vi "Lab Panel V4.90.vi"() -> ()   [LabVIEW 2013] (continued)
                n1776 = property on="O/I  LAB04-2" class="Bool (strict)"("DisabledEnum"=w3325) -> ()  [unwired: 2 in, 2 out]
                n1777 = property on="O/I  LAB03-2" class="Bool (strict)"("DisabledEnum"=w3327) -> ()  [unwired: 2 in, 2 out]
                n1778 = Not(x=w3332) -> (.not. x?=w3333:bool)
                n1779 = Not(x=w3331) -> (.not. x?=w3334:bool)
                n1780 = Not(x=w3330) -> (.not. x?=w3335:bool)
                n1781 = property on="RESULT LAB05-2" class="Bool (strict)"("Visible"=w3333) -> ()  [unwired: 2 in, 2 out]
                n1782 = property on="RESULT LAB05-1" class="Bool (strict)"("Visible"=w3334) -> ()  [unwired: 2 in, 2 out]
                n1783 = Not(x=w3329) -> (.not. x?=w3336:bool)
                n1784 = property on="RESULT LAB04-2" class="Bool (strict)"("Visible"=w3335) -> ()  [unwired: 2 in, 2 out]
                n1785 = Not(x=w3328) -> (.not. x?=w3337:bool)
                n1786 = property on="RESULT LAB04-1" class="Bool (strict)"("Visible"=w3336) -> ()  [unwired: 2 in, 2 out]
                n1787 = property on="RESULT LAB03-2" class="Bool (strict)"("Visible"=w3337) -> ()  [unwired: 2 in, 2 out]
              }
              frame #2 {
                # "disable calibrate if any test running"
                n1788 = Or(x=w3360, y=w3359) -> (x .or. y?=w3353:bool)
                n1789 = Or(x=w3362, y=w3361) -> (x .or. y?=w3355:bool)
                n1790 = Or(x=w3366, y=w3365) -> (x .or. y?=w3357:bool)
                n1791 = Or(x=w3364, y=w3363) -> (x .or. y?=w3356:bool)
                n1792 = Or(x=w3368, y=w3367) -> (x .or. y?=w3358:bool)
                n1793 = Or(x=w3356, y=w3355) -> (x .or. y?=w3354:bool)
                n1794 = Or(x=w3358, y=w3357) -> (x .or. y?=w3352:bool)
                n1795 = Or(x=w3354, y=w3353) -> (x .or. y?=w3351:bool)
                n1796 = Or(x=w3352, y=w3351) -> (x .or. y?=w3350:bool)
                n1797 = case shown="False" w3350 {
                  tunnel: [0 2] -> w3349
                  frame False {
                  }
                  frame True {
                  }
                }
                n1798 = property on="JIG TEST" class="Clust (strict)"("DisabledEnum"=w3349) -> ()  [unwired: 2 in, 2 out]
                n1799 = property on="Network Directory" class="Path"("DisabledEnum"=w3349) -> ()  [unwired: 2 in, 2 out]
                n1800 = property on="MAIL SETTINGS" class="Clust (strict)"("DisabledEnum"=w3349) -> ()  [unwired: 2 in, 2 out]
                n1801 = property on="SET (cal)" class="Bool (strict)"("DisabledEnum"=w3349) -> ()  [unwired: 2 in, 2 out]
                n1802 = property on="ADMIN" class="Bool (strict)"("DisabledEnum"=0) -> ()  [unwired: 2 in, 2 out]
              }
            }
          }
          frame #8 {
            # "drive jigs"
            n1803 = stacked-sequence {
              frame #0 {
                # "jig on"
                n1804 = local read "jig cycle"() -> (w3376:dbl)
                n1805 = property on="JIG TEST" class="Clust (strict)"() -> ("DisabledEnum"=w3373:T16)  [unwired: 2 in, 2 out]
                n1806 = Equal?(x=w3373, y=2) -> (x = y?=w3372:bool)
                n1807 = Equal?(x=w3376, y=0) -> (x = y?=w3374:bool)
                n1808 = And(x=w3374, y=w3372) -> (x .and. y?=w3371:bool)
                n1809 = case shown="True" w3371 {
                  frame False {
                  }
                  frame True {
                    n1810 = local read "run lab01-1"() -> (w3387:bool)
                    n1811 = local read "run lab01-2"() -> (w3386:bool)
                    n1812 = local read "run lab02-1"() -> (w3385:bool)
                    n1813 = local read "run lab02-2"() -> (w3384:bool)
                    n1814 = local read "run lab03-1"() -> (w3383:bool)
                    n1815 = local read "run lab03-2"() -> (w3382:bool)
                    n1816 = local read "run lab04-1"() -> (w3381:bool)
                    n1817 = local read "run lab04-2"() -> (w3380:bool)
                    n1818 = local read "run lab05-1"() -> (w3379:bool)
                    n1819 = local read "run lab05-2"() -> (w3378:bool)
                    n1820 = local write "JIG LAB03-2"(w3382) -> ()
                    n1821 = local write "JIG LAB01-1"(w3387) -> ()
                    n1822 = local write "JIG LAB01-2"(w3386) -> ()
                    n1823 = local write "JIG LAB02-1"(w3385) -> ()
                    n1824 = local write "JIG LAB02-2"(w3384) -> ()
                    n1825 = local write "JIG LAB03-1"(w3383) -> ()
                    n1826 = local write "JIG LAB04-1"(w3381) -> ()
                    n1827 = local write "JIG LAB04-2"(w3380) -> ()
                    n1828 = local write "JIG LAB05-1"(w3379) -> ()
                    n1829 = local write "JIG LAB05-2"(w3378) -> ()
                  }
                }
              }
              frame #1 {
                # "jig off"
                n1830 = local read "jig cycle"() -> (w3394:dbl)
                n1831 = local read "on loops"() -> (w3393:dbl)
                n1832 = property on="JIG TEST" class="Clust (strict)"() -> ("DisabledEnum"=w3392:T16)  [unwired: 2 in, 2 out]
                n1833 = Equal?(x=w3392, y=2) -> (x = y?=w3390:bool)
                n1834 = Equal?(x=w3394, y=w3393) -> (x = y?=w3389:bool)
                n1835 = And(x=w3389, y=w3390) -> (x .and. y?=w3388:bool)
                n1836 = case shown="True" w3388 {
                  frame False {
                  }
                  frame True {
                    w3445 = FALSE
                    w3446 = TRUE
                    w3444 = 2
                    n1837 = local read "SELECT LAB05-2"() -> (w3435:T3)
                    n1838 = local read "SELECT LAB04-2"() -> (w3437:T3)
                    n1839 = local read "SELECT LAB04-1"() -> (w3438:T3)
                    n1840 = local read "SELECT LAB05-1"() -> (w3436:T3)
                    n1841 = local read "SELECT LAB03-2"() -> (w3439:T3)
                    n1842 = local read "SELECT LAB02-1"() -> (w3442:T3)
                    n1843 = local read "SELECT LAB03-1"() -> (w3440:T3)
                    n1844 = local read "SELECT LAB02-2"() -> (w3441:T3)
                    n1845 = local read "SELECT LAB01-2"() -> (w3443:T3)
                    n1846 = local read "run lab05-1"() -> (w3405:bool)
                    n1847 = local read "run lab05-2"() -> (w3404:bool)
                    n1848 = local read "SELECT LAB01-1"() -> (w3447:T3)
                    n1849 = local read "run lab04-2"() -> (w3406:bool)
                    n1850 = local read "run lab04-1"() -> (w3407:bool)
                    n1851 = local read "run lab01-1"() -> (w3423:bool)
                    n1852 = local read "run lab01-2"() -> (w3412:bool)
                    n1853 = local read "run lab03-2"() -> (w3408:bool)
                    n1854 = local read "run lab03-1"() -> (w3409:bool)
                    n1855 = local read "run lab02-1"() -> (w3411:bool)
                    n1856 = local read "run lab02-2"() -> (w3410:bool)
                    n1857 = Equal?(x=w3444, y=w3440) -> (x = y?=w3418:bool)
                    n1858 = Equal?(x=w3444, y=w3439) -> (x = y?=w3417:bool)
                    n1859 = Equal?(x=w3444, y=w3438) -> (x = y?=w3416:bool)
                    n1860 = Equal?(x=w3444, y=w3437) -> (x = y?=w3415:bool)
                    n1861 = Equal?(x=w3444, y=w3436) -> (x = y?=w3414:bool)
                    n1862 = Equal?(x=w3444, y=w3435) -> (x = y?=w3413:bool)
                    n1863 = Equal?(x=w3444, y=w3447) -> (x = y?=w3424:bool)
                    n1864 = Equal?(x=w3444, y=w3442) -> (x = y?=w3420:bool)
                    n1865 = Equal?(x=w3444, y=w3441) -> (x = y?=w3419:bool)
                    n1866 = Equal?(x=w3444, y=w3443) -> (x = y?=w3421:bool)
                    n1867 = And(x=w3415, y=w3406) -> (x .and. y?=w3397:bool)
                    n1868 = And(x=w3418, y=w3409) -> (x .and. y?=w3400:bool)
                    n1869 = And(x=w3416, y=w3407) -> (x .and. y?=w3398:bool)
                    n1870 = And(x=w3413, y=w3404) -> (x .and. y?=w3395:bool)
                    n1871 = And(x=w3419, y=w3410) -> (x .and. y?=w3401:bool)
                    n1872 = And(x=w3417, y=w3408) -> (x .and. y?=w3399:bool)
                    n1873 = And(x=w3414, y=w3405) -> (x .and. y?=w3396:bool)
                    n1874 = And(x=w3421, y=w3412) -> (x .and. y?=w3403:bool)
                    n1875 = And(x=w3424, y=w3423) -> (x .and. y?=w3422:bool)
                    n1876 = And(x=w3420, y=w3411) -> (x .and. y?=w3402:bool)
                    n1877 = Select(t=w3446, s=w3422, f=w3445) -> (s? t:f=w3425:bool)
                    n1878 = Select(t=w3446, s=w3403, f=w3445) -> (s? t:f=w3426:bool)
                    n1879 = Select(t=w3446, s=w3402, f=w3445) -> (s? t:f=w3427:bool)
                    n1880 = Select(t=w3446, s=w3401, f=w3445) -> (s? t:f=w3428:bool)
                    n1881 = Select(t=w3446, s=w3400, f=w3445) -> (s? t:f=w3429:bool)
                    n1882 = Select(t=w3446, s=w3399, f=w3445) -> (s? t:f=w3430:bool)
                    n1883 = Select(t=w3446, s=w3398, f=w3445) -> (s? t:f=w3431:bool)
                    n1884 = Select(t=w3446, s=w3397, f=w3445) -> (s? t:f=w3432:bool)
                    n1885 = Select(t=w3446, s=w3396, f=w3445) -> (s? t:f=w3433:bool)
                    n1886 = Select(t=w3446, s=w3395, f=w3445) -> (s? t:f=w3434:bool)
                    n1887 = local write "JIG LAB03-2"(w3430) -> ()
                    n1888 = local write "JIG LAB02-1"(w3427) -> ()
                    n1889 = local write "JIG LAB02-2"(w3428) -> ()
                    n1890 = local write "JIG LAB01-2"(w3426) -> ()
                    n1891 = local write "JIG LAB03-1"(w3429) -> ()
                    n1892 = local write "JIG LAB01-1"(w3425) -> ()
                    n1893 = local write "JIG LAB05-2"(w3434) -> ()
                    n1894 = local write "JIG LAB04-1"(w3431) -> ()
                    n1895 = local write "JIG LAB05-1"(w3433) -> ()
                    n1896 = local write "JIG LAB04-2"(w3432) -> ()
                  }
                }
              }
            }
          }
          frame #9 {
            # "enable  jig test output if no test busy"
            n1897 = property on="JIG TEST" class="Clust (strict)"() -> ("DisabledEnum"=w3450:T16)  [unwired: 2 in, 2 out]
            n1898 = Equal?(x=w3450, y=0) -> (x = y?=w3448:bool)
            n1899 = case shown="True" w3448 {
              frame False {
              }
              frame True {
                n1900 = local read "JIG TEST"() -> (w3461:T10)
                n1901 = Unbundle(w3461) -> ("LAB01-1"=w3460:bool, "LAB01-2"=w3459:bool, "LAB02-1"=w3458:bool, "LAB02-2"=w3457:bool, "LAB03-1"=w3456:bool, "LAB03-2"=w3455:bool, "LAB04-1"=w3454:bool, "LAB04-2"=w3453:bool, "LAB05-1"=w3452:bool, "LAB05-2"=w3451:bool)
                n1902 = local write "JIG LAB05-1"(w3452) -> ()
                n1903 = local write "JIG LAB05-2"(w3451) -> ()
                n1904 = local write "JIG LAB04-1"(w3454) -> ()
                n1905 = local write "JIG LAB04-2"(w3453) -> ()
                n1906 = local write "JIG LAB03-2"(w3455) -> ()
                n1907 = local write "JIG LAB01-1"(w3460) -> ()
                n1908 = local write "JIG LAB02-1"(w3458) -> ()
                n1909 = local write "JIG LAB03-1"(w3456) -> ()
                n1910 = local write "JIG LAB01-2"(w3459) -> ()
                n1911 = local write "JIG LAB02-2"(w3457) -> ()
              }
            }
          }
          frame #10 {
            # "drive digital output"
            n1912 = local read "O/I  LAB05-2"() -> (w3468:bool)
            n1913 = local read "O/I  LAB05-1"() -> (w3470:bool)
            n1914 = local read "JIG LAB05-2"() -> (w3467:bool)
            n1915 = local read "O/I  LAB04-2"() -> (w3472:bool)
            n1916 = local read "JIG LAB05-1"() -> (w3469:bool)
            n1917 = local read "JIG LAB04-2"() -> (w3471:bool)
            n1918 = local read "O/I  LAB03-1"() -> (w3477:bool)
            n1919 = local read "O/I  LAB04-1"() -> (w3473:bool)
            n1920 = local read "O/I  LAB02-1"() -> (w3481:bool)
            n1921 = local read "O/I  LAB02-2"() -> (w3479:bool)
            n1922 = local read "O/I  LAB03-2"() -> (w3475:bool)
            n1923 = local read "JIG LAB04-1"() -> (w3466:bool)
            n1924 = local read "JIG LAB03-2"() -> (w3474:bool)
            n1925 = local read "O/I  LAB01-2"() -> (w3483:bool)
            n1926 = local read "JIG LAB02-1"() -> (w3480:bool)
            n1927 = local read "JIG LAB02-2"() -> (w3478:bool)
            n1928 = local read "JIG LAB03-1"() -> (w3476:bool)
            n1929 = local read "O/I  LAB01-1"() -> (w3485:bool)
            n1930 = local read "JIG LAB01-2"() -> (w3482:bool)
            n1931 = local read "JIG LAB01-1"() -> (w3484:bool)
            n1932 = Build Array(w3472, w3471, w3470, w3469, w3468, w3467) -> (w3463:bool[])
            n1933 = Build Array(w3478, w3477, w3476, w3475, w3474, w3473, w3466) -> (w3464:bool[])
            n1934 = Build Array(w3485, w3484, w3483, w3482, w3481, w3480, w3479) -> (w3465:bool[])
            n1935 = local read "simulate"() -> (w3462:bool)
            n1936 = case shown="False" w3462 {
              tunnel: w3465 -> [w3488 _]
              tunnel: w3464 -> [w3487 _]
              tunnel: w3463 -> [w3486 _]
              frame False {
                n1937 = call "sub vi - Drive Relays All v6.vi"("Array #2"=w3486, "Array #1"=w3487, "Array #0"=w3488) -> ()  [unwired: 8 in, 1 out]
              }
              frame True {
              }
            }
          }
          frame #11 {
            # "get analog values"
            n1938 = local read "on loops"() -> (w3495:dbl)
            n1939 = local read "jig cycle"() -> (w3492:dbl)
            n1940 = Add(x=w3495, y=1) -> (x+y=w3493:dbl)
            n1941 = Equal?(x=w3492, y=1) -> (x = y?=w3489:bool)
            n1942 = Equal?(x=w3492, y=w3493) -> (x = y?=w3491:bool)
            n1943 = Or(x=w3489, y=w3491) -> (x .or. y?=w3490:bool)
            n1944 = global write "Global display 3.vi" "cycle O/F"(w3489) -> ()
            n1945 = case shown="True" w3490 {
              tunnel: w3489 -> [_ w3498]
              frame False {
              }
              frame True {
                n1946 = local read "simulate"() -> (w3501:bool)
                n1947 = case shown="True" w3501 {
                  tunnel: [w3511 errorcluster[] [] ("array ERROR")] -> w3509
                  tunnel: [w3518 0.3 ("Analog loop time")] -> w3508
                  tunnel: [w3517 dynamicdata[] [] ("array GRAPH")] -> w3507
                  tunnel: [w3516 w3522] -> w3506
                  tunnel: [w3515 w3522] -> w3505
                  tunnel: [w3514 w3522] -> w3504
                  tunnel: [w3513 w3522] -> w3503
                  tunnel: [w3512 w3522] -> w3502
                  tunnel: w3498 -> [_ w3526]
                  tunnel: [w3510 2.92] -> w3497
                  frame False {
                    n1948 = call "sub vi - Read Analog All v9.11.vi"() -> ("Analog loop time"=w3518:dbl, "array GRAPH"=w3517:dynamicdata[], "LAB01"=w3516:T26, "LAB02"=w3515:T27, "LAB03"=w3514:T28, "LAB04"=w3513:T29, "deg C"=w3510:dbl, "Any Error"=w3511:bool, "LAB05"=w3512:T30)  [unwired: 7 in]
                  }
                  frame True {
                    n1949 = local read "ON amps"() -> (w3519:dbl)
                    n1950 = local read "OFF amps"() -> (w3520:dbl)
                    n1951 = local read "VOLTS"() -> (w3524:dbl)
                    n1952 = local read "PF"() -> (w3523:dbl)
                    n1953 = Select(t=w3519, s=w3526, f=w3520) -> (s? t:f=w3525:dbl)
                    n1954 = Bundle("OFF amps"=w3525, "VOLTS"=w3524, "PF"=w3523, "OFF amps"=w3525, "VOLTS"=w3524, "PF"=w3523) -> (w3522:T31)  [unwired: 1 in]
                  }
                }
                n1955 = local read "simulate"() -> (w3500:bool)
                n1956 = stacked-sequence {
                  tunnel: w3509 -> [w3534 _ _ _ _ _ _]
                  tunnel: w3508 -> [w3533 _ _ _ _ _ _]
                  tunnel: w3507 -> [w3530 _ _ _ _ _ _]
                  tunnel: w3506 -> [_ w3581 _ _ _ _ _]
                  tunnel: w3505 -> [_ _ w3588 _ _ _ _]
                  tunnel: w3504 -> [_ _ _ w3617 _ _ _]
                  tunnel: w3503 -> [_ _ _ _ w3644 _ _]
                  tunnel: w3502 -> [_ _ _ _ _ w3673 _]
                  tunnel: w3500 -> [_ w3559 w3587 w3615 w3643 w3671 w3697]
                  tunnel: T14 {"1  (A) cal"=1.0, "1 (V) cal"=1.0, "1 (PF) cal"=1.0, "1 (TL) cal"=1.0, "1 (TN) cal"=1.0, "2 (A) cal"=1.0, "2 (V) cal"=1.0, "2 (PF) cal"=1.0, "2 (TL) cal"=1.0, "2 (TN) cal"=1.0} ("CAL LAB01") -> [_ w3558 w3586 w3614 w3642 w3670 _]
                  tunnel: w3497 -> [_ _ _ _ _ _ w3696]
                  frame #0 {
                    n1957 = local write "AI"(TRUE) -> ()
                    n1958 = global write "Global 1.vi" "RATE(Hz)"("RATE (Hz)") -> ()
                    n1959 = global write "Global 1.vi" "SAMPLES"("SAMPLES") -> ()
                    n1960 = Index Array(array=w3530, index=6) -> (element=→"LAB04-1 (GRAPH)":dynamicdata)
                    n1961 = Index Array(array=w3530, index=7) -> (element=→"LAB04-2 (GRAPH)":dynamicdata)
                    n1962 = Index Array(array=w3530, index=9) -> (element=→"LAB05-2 (GRAPH)":dynamicdata)
                    n1963 = Index Array(array=w3530, index=8) -> (element=→"LAB05-1 (GRAPH)":dynamicdata)
                    n1964 = Index Array(array=w3530, index=5) -> (element=→"LAB03-2 (GRAPH)":dynamicdata)
                    n1965 = Index Array(array=w3530, index=0) -> (element=→"LAB01-1 (GRAPH)":dynamicdata)
                    n1966 = Index Array(array=w3530, index=1) -> (element=→"LAB01-2 (GRAPH)":dynamicdata)
                    n1967 = Index Array(array=w3530, index=2) -> (element=→"LAB02-1 (GRAPH)":dynamicdata)
                    n1968 = Index Array(array=w3530, index=3) -> (element=→"LAB02-2 (GRAPH)":dynamicdata)
                    n1969 = Index Array(array=w3530, index=4) -> (element=→"LAB03-1 (GRAPH)":dynamicdata)
                    "AI loop time" <- w3533
                    "Analog Error Array" <- w3534
                  }
                  frame #1 {
                    n1970 = case shown="False" w3559 {
                      tunnel: [w3582 w3583] -> w3580
                      tunnel: w3558 -> [_ w3583]
                      frame False {
                        n1971 = local read "CAL LAB01"() -> (w3582:T14)
                      }
                      frame True {
                      }
                    }
                    n1972 = Unbundle By Name(w3581) -> ("OFF amps"=w3579:dbl, "VOLTS"=w3578:dbl, "PF"=w3577:dbl, "OFF amps"=w3576:dbl, "VOLTS"=w3575:dbl, "PF"=w3574:dbl)
                    n1973 = Unbundle By Name(w3580) -> ("1  (A) cal"=w3573:dbl, "1 (V) cal"=w3572:dbl, "1 (PF) cal"=w3571:dbl, "2 (A) cal"=w3570:dbl, "2 (V) cal"=w3569:dbl, "2 (PF) cal"=w3568:dbl)  [unwired: 4 out]
                    n1974 = Multiply(x=w3579, y=w3573) -> (x*y=w3566:dbl)
                    n1975 = Multiply(x=w3578, y=w3572) -> (x*y=w3565:dbl)
                    n1976 = Multiply(x=w3577, y=w3571) -> (x*y=w3564:dbl)
                    n1977 = Multiply(x=w3576, y=w3570) -> (x*y=w3562:dbl)
                    n1978 = Multiply(x=w3575, y=w3569) -> (x*y=w3561:dbl)
                    n1979 = Multiply(x=w3574, y=w3568) -> (x*y=w3560:dbl)
                    n1980 = local read "SIG LAB01-1"() -> (w3567:T2)
                    n1981 = local read "SIG LAB01-2"() -> (w3563:T2)
                    n1982 = Bundle By Name(cluster=w3567, "AMPS"=w3566, "VOLTS"=w3565, "PF"=w3564) -> (w3557:T2)
                    n1983 = Bundle By Name(cluster=w3563, "AMPS"=w3562, "VOLTS"=w3561, "PF"=w3560) -> (w3556:T2)
                    n1984 = global write "Global display 1.vi" "SIG LAB01-2"(w3556) -> ()
                    n1985 = global write "Global display 1.vi" "SIG LAB01-1"(w3557) -> ()
                    n1986 = local write "SIG LAB01-2"(w3556) -> ()
                    n1987 = local write "SIG LAB01-1"(w3557) -> ()
                  }
                  frame #2 {
                    n1988 = Unbundle By Name(w3588) -> ("OFF amps"=w3608:dbl, "VOLTS"=w3607:dbl, "PF"=w3606:dbl, "OFF amps"=w3605:dbl, "VOLTS"=w3604:dbl, "PF"=w3603:dbl)
                    n1989 = case shown="True" w3587 {
                      tunnel: [w3610 w3611] -> w3609
                      tunnel: w3586 -> [_ w3611]
                      frame False {
                        n1990 = local read "CAL LAB02"() -> (w3610:T15)
                      }
                      frame True {
                      }
                    }
                    n1991 = Unbundle By Name(w3609) -> ("1  (A) cal"=w3602:dbl, "1 (V) cal"=w3601:dbl, "1 (PF) cal"=w3600:dbl, "2 (A) cal"=w3599:dbl, "2 (V) cal"=w3598:dbl, "2 (PF) cal"=w3597:dbl)  [unwired: 4 out]
                    n1992 = Multiply(x=w3608, y=w3602) -> (x*y=w3595:dbl)
                    n1993 = Multiply(x=w3607, y=w3601) -> (x*y=w3594:dbl)
                    n1994 = Multiply(x=w3606, y=w3600) -> (x*y=w3593:dbl)
                    n1995 = Multiply(x=w3605, y=w3599) -> (x*y=w3591:dbl)
                    n1996 = Multiply(x=w3604, y=w3598) -> (x*y=w3590:dbl)
                    n1997 = Multiply(x=w3603, y=w3597) -> (x*y=w3589:dbl)
                    n1998 = local read "SIG LAB02-1"() -> (w3596:T2)
                    n1999 = local read "SIG LAB02-2"() -> (w3592:T2)
                    n2000 = Bundle By Name(cluster=w3596, "AMPS"=w3595, "VOLTS"=w3594, "PF"=w3593) -> (w3585:T2)
                    n2001 = Bundle By Name(cluster=w3592, "AMPS"=w3591, "VOLTS"=w3590, "PF"=w3589) -> (w3584:T2)
                    n2002 = global write "Global display 1.vi" "SIG LAB02-1"(w3585) -> ()
                    n2003 = local write "SIG LAB02-2"(w3584) -> ()
                    n2004 = global write "Global display 1.vi" "SIG LAB02-2"(w3584) -> ()
                    n2005 = local write "SIG LAB02-1"(w3585) -> ()
                  }
                  frame #3 {
                    n2006 = Unbundle By Name(w3617) -> ("OFF amps"=w3636:dbl, "VOLTS"=w3635:dbl, "PF"=w3634:dbl, "OFF amps"=w3633:dbl, "VOLTS"=w3632:dbl, "PF"=w3631:dbl)
                    n2007 = case shown="True" w3615 {
                      tunnel: [w3638 w3639] -> w3637
                      tunnel: w3614 -> [_ w3639]
                      frame False {
                        n2008 = local read "CAL LAB03"() -> (w3638:T14)
                      }
                      frame True {
                      }
                    }
                    n2009 = Unbundle By Name(w3637) -> ("1  (A) cal"=w3630:dbl, "1 (V) cal"=w3629:dbl, "1 (PF) cal"=w3628:dbl, "2 (A) cal"=w3627:dbl, "2 (V) cal"=w3626:dbl, "2 (PF) cal"=w3625:dbl)  [unwired: 4 out]
                    n2010 = Multiply(x=w3636, y=w3630) -> (x*y=w3623:dbl)
                    n2011 = Multiply(x=w3635, y=w3629) -> (x*y=w3616:dbl)
                    n2012 = Multiply(x=w3634, y=w3628) -> (x*y=w3622:dbl)
                    n2013 = Multiply(x=w3633, y=w3627) -> (x*y=w3620:dbl)
                    n2014 = Multiply(x=w3632, y=w3626) -> (x*y=w3619:dbl)
                    n2015 = Multiply(x=w3631, y=w3625) -> (x*y=w3618:dbl)
                    n2016 = local read "SIG LAB03-1"() -> (w3624:T2)
                    n2017 = local read "SIG LAB03-2"() -> (w3621:T2)
                    n2018 = Bundle By Name(cluster=w3624, "AMPS"=w3623, "VOLTS"=w3616, "PF"=w3622) -> (w3613:T2)
                    n2019 = Bundle By Name(cluster=w3621, "AMPS"=w3620, "VOLTS"=w3619, "PF"=w3618) -> (w3612:T2)
                    n2020 = global write "Global display 1.vi" "SIG LAB03-1"(w3613) -> ()
                    n2021 = global write "Global display 1.vi" "SIG LAB03-2"(w3612) -> ()
                    n2022 = local write "SIG LAB03-2"(w3612) -> ()
                    n2023 = local write "SIG LAB03-1"(w3613) -> ()
                  }
                  frame #4 {
                    n2024 = Unbundle By Name(w3644) -> ("OFF amps"=w3664:dbl, "VOLTS"=w3663:dbl, "PF"=w3662:dbl, "OFF amps"=w3661:dbl, "VOLTS"=w3660:dbl, "PF"=w3659:dbl)
                    n2025 = case shown="False" w3643 {
                      tunnel: [w3666 w3667] -> w3665
                      tunnel: w3642 -> [_ w3667]
                      frame False {
                        n2026 = local read "CAL LAB04"() -> (w3666:T14)
                      }
                      frame True {
                      }
                    }
                    n2027 = Unbundle By Name(w3665) -> ("1  (A) cal"=w3658:dbl, "1 (V) cal"=w3657:dbl, "1 (PF) cal"=w3656:dbl, "2 (A) cal"=w3655:dbl, "2 (V) cal"=w3654:dbl, "2 (PF) cal"=w3653:dbl)  [unwired: 4 out]
                    n2028 = Multiply(x=w3664, y=w3658) -> (x*y=w3651:dbl)
                    n2029 = Multiply(x=w3663, y=w3657) -> (x*y=w3650:dbl)
                    n2030 = Multiply(x=w3662, y=w3656) -> (x*y=w3649:dbl)
                    n2031 = Multiply(x=w3661, y=w3655) -> (x*y=w3647:dbl)
                    n2032 = Multiply(x=w3660, y=w3654) -> (x*y=w3646:dbl)
                    n2033 = Multiply(x=w3659, y=w3653) -> (x*y=w3645:dbl)
                    n2034 = local read "SIG LAB04-1"() -> (w3652:T2)
                    n2035 = local read "SIG LAB04-2"() -> (w3648:T2)
                    n2036 = Bundle By Name(cluster=w3652, "AMPS"=w3651, "VOLTS"=w3650, "PF"=w3649) -> (w3641:T2)
                    n2037 = Bundle By Name(cluster=w3648, "AMPS"=w3647, "VOLTS"=w3646, "PF"=w3645) -> (w3640:T2)
                    n2038 = global write "Global display 1.vi" "SIG LAB04-2"(w3640) -> ()
                    n2039 = global write "Global display 1.vi" "SIG LAB04-1"(w3641) -> ()
                    n2040 = local write "SIG LAB04-2"(w3640) -> ()
                    n2041 = local write "SIG LAB04-1"(w3641) -> ()
                  }
                  frame #5 {
                    n2042 = Unbundle By Name(w3673) -> ("OFF amps"=w3692:dbl, "VOLTS"=w3672:dbl, "PF"=w3691:dbl, "OFF amps"=w3690:dbl, "VOLTS"=w3689:dbl, "PF"=w3688:dbl)
                    n2043 = case shown="False" w3671 {
                      tunnel: [w3694 w3695] -> w3693
                      tunnel: w3670 -> [_ w3695]
                      frame False {
                        n2044 = local read "CAL LAB05"() -> (w3694:T14)
                      }
                      frame True {
                      }
                    }
                    n2045 = Unbundle By Name(w3693) -> ("1  (A) cal"=w3687:dbl, "1 (V) cal"=w3686:dbl, "1 (PF) cal"=w3685:dbl, "2 (A) cal"=w3684:dbl, "2 (V) cal"=w3683:dbl, "2 (PF) cal"=w3682:dbl)  [unwired: 4 out]
                    n2046 = Multiply(x=w3692, y=w3687) -> (x*y=w3680:dbl)
                    n2047 = Multiply(x=w3672, y=w3686) -> (x*y=w3679:dbl)
                    n2048 = Multiply(x=w3691, y=w3685) -> (x*y=w3678:dbl)
                    n2049 = Multiply(x=w3690, y=w3684) -> (x*y=w3676:dbl)
                    n2050 = Multiply(x=w3689, y=w3683) -> (x*y=w3675:dbl)
                    n2051 = Multiply(x=w3688, y=w3682) -> (x*y=w3674:dbl)
                    n2052 = local read "SIG LAB05-1"() -> (w3681:T2)
                    n2053 = local read "SIG LAB05-2"() -> (w3677:T2)
                    n2054 = Bundle By Name(cluster=w3681, "AMPS"=w3680, "VOLTS"=w3679, "PF"=w3678) -> (w3669:T2)
                    n2055 = Bundle By Name(cluster=w3677, "AMPS"=w3676, "VOLTS"=w3675, "PF"=w3674) -> (w3668:T2)
                    n2056 = global write "Global display 1.vi" "SIG LAB05-1"(w3669) -> ()
                    n2057 = global write "Global display 1.vi" "SIG LAB05-2"(w3668) -> ()
                    n2058 = local write "SIG LAB05-2"(w3668) -> ()
                    n2059 = local write "SIG LAB05-1"(w3669) -> ()
                  }
                  frame #6 {
                    # "update ambient referance temperature"
                    n2060 = case shown="False" w3697 {
                      tunnel: [w3700 100.0] -> w3699
                      frame False {
                        n2061 = local read "TEMP REF cal"() -> (w3700:dbl)
                      }
                      frame True {
                      }
                    }
                    n2062 = local read "Panel #"() -> (w3698:dbl)
                    n2063 = case shown="1" w3698 {
                      tunnel: w3699 -> [_ w3706]
                      tunnel: w3696 -> [_ w3705]
                      frame 0, Default {
                      }
                      frame 1 {
                        n2064 = Multiply(x=w3706, y=w3705) -> (x*y=w3704:dbl)
                        n2065 = Subtract(x=w3704, y=272) -> (x-y=w3702:dbl)
                        "Amb Ref" <- w3702
                        n2066 = local write "Ref deg C"(w3702) -> ()
                      }
                    }
                    "deg C (volts)" <- w3696
                  }
                }
              }
            }
          }
          frame #12 {
            # "save test data to file"
            n2067 = Get Date/Time In Seconds() -> (seconds since 1Jan1904=w3707:timestamp)
            "File Time Stamp" <- w3707
            n2068 = local read "on loops"() -> (w3726:dbl)
            n2069 = local read "jig cycle"() -> (w3723:dbl)
            n2070 = Format Date/Time String(time format string (%c)="%H:%M%:%S", seconds (now)=w3707) -> (date/time string=w3711:string)  [unwired: 1 in]
            n2071 = Add(x=w3726, y=2) -> (x+y=w3724:dbl)
            n2072 = Build Array(w3711) -> (w3710:string[])
            n2073 = Equal?(x=w3723, y=1) -> (x = y?=w3709:bool)
            n2074 = Equal?(x=w3723, y=w3724) -> (x = y?=w3708:bool)
            n2075 = stacked-sequence {
              tunnel: w3722 -> [w3732 _ _ _ _ _ _ _ _ _]
              tunnel: w3721 -> [_ w3808 _ _ _ _ _ _ _ _]
              tunnel: w3720 -> [_ _ w3888 _ _ _ _ _ _ _]
              tunnel: w3719 -> [_ _ _ w3968 _ _ _ _ _ _]
              tunnel: w3718 -> [_ _ _ _ w4048 _ _ _ _ _]
              tunnel: w3717 -> [_ _ _ _ _ w4128 _ _ _ _]
              tunnel: w3716 -> [_ _ _ _ _ _ w4208 _ _ _]
              tunnel: w3715 -> [_ _ _ _ _ _ _ w4288 _ _]
              tunnel: w3714 -> [_ _ _ _ _ _ _ _ w4368 _]
              tunnel: w3713 -> [_ _ _ _ _ _ _ _ _ w4448]
              tunnel: w3710 -> [w3731 w3812 w3892 w3972 w4052 w4132 w4212 w4292 w4372 w4452]
              tunnel: w3709 -> [w3730 w3811 w3891 w3971 w4051 w4131 w4211 w4291 w4371 w4451]
              tunnel: w3708 -> [w3729 w3810 w3890 w3970 w4050 w4130 w4210 w4290 w4370 w4450]
              tunnel: w3707 -> [w3728 w3809 w3889 w3969 w4049 w4129 w4209 w4289 w4369 w4449]
              frame #0 {
                n2076 = case shown="True" w3732 {
                  tunnel: w3731 -> [_ w3737]
                  tunnel: w3730 -> [_ w3736]
                  tunnel: w3729 -> [_ w3734]
                  tunnel: w3728 -> [_ w3733]
                  frame False {
                  }
                  frame True {
                    n2077 = local read "DISP LAB01-1"() -> (w3738:T4)
                    n2078 = local read "SIG LAB01-1"() -> (w3739:T2)
                    n2079 = local read "ON L01-1"() -> (w3735:cluster{"amps":dbl, "volts":dbl, "pf":dbl})
                    n2080 = Unbundle(w3739) -> ("AMPS"=w3745:dbl, "VOLTS"=w3743:dbl, "PF"=w3742:dbl, "Tmp Live"=w3741:dbl, "Tmp Neut"=w3744:dbl)
                    n2081 = Unbundle(w3738) -> ("CYCLE"=w3740:dbl)  [unwired: 2 out]
                    n2082 = stacked-sequence {
                      tunnel: w3745 -> [w3749 w3768]
                      tunnel: w3744 -> [_ w3767]
                      tunnel: w3743 -> [w3748 w3766]
                      tunnel: w3742 -> [w3747 w3765]
                      tunnel: w3741 -> [_ w3764]
                      tunnel: w3740 -> [_ w3763]
                      tunnel: w3737 -> [_ w3762]
                      tunnel: w3736 -> [w3750 _]
                      tunnel: w3735 -> [w3746 w3760]
                      tunnel: w3734 -> [_ w3761]
                      tunnel: w3733 -> [_ w3756]
                      frame #0 {
                        n2083 = case shown="True" w3750 {
                          tunnel: w3749 -> [_ w3755]
                          tunnel: w3748 -> [_ w3754]
                          tunnel: w3747 -> [_ w3753]
                          tunnel: w3746 -> [_ w3751]
                          frame False {
                          }
                          frame True {
                            n2084 = Bundle(cluster=w3751, "amps"=w3755, "volts"=w3754, "pf"=w3753) -> (w3752:cluster{"amps":dbl, "volts":dbl, "pf":dbl})
                            n2085 = local write "ON L01-1"(w3752) -> ()
                          }
                        }
                      }
                      frame #1 {
                        n2086 = Unbundle(w3760) -> ("amps"=w3759:dbl, "volts"=w3758:dbl, "pf"=w3757:dbl)
                        n2087 = case shown="True" w3761 {
                          tunnel: w3768 -> [_ w3769]
                          tunnel: w3767 -> [_ w3807]
                          tunnel: w3766 -> [_ _]
                          tunnel: w3765 -> [_ _]
                          tunnel: w3764 -> [_ w3806]
                          tunnel: w3763 -> [_ w3805]
                          tunnel: w3762 -> [_ w3773]
                          tunnel: w3759 -> [_ w3770]
                          tunnel: w3758 -> [_ w3802]
                          tunnel: w3757 -> [_ w3801]
                          tunnel: w3756 -> [_ w3771]
                          frame False {
                          }
                          frame True {
                            n2088 = local read "TDMS LAB01-1"() -> (w3804:refnum<k34>)
                            n2089 = Build Array(w3802) -> (w3798:dbl[])
                            n2090 = Build Array(w3801) -> (w3797:dbl[])
                            n2091 = Build Array(w3806) -> (w3796:dbl[])
                            n2092 = Build Array(w3807) -> (w3795:dbl[])
                            n2093 = Build Array(w3770) -> (w3800:dbl[])
                            n2094 = Build Array(w3769) -> (w3799:dbl[])
                            n2095 = Build Array(w3805) -> (w3794:dbl[])
                            n2096 = Build Array("AMPS ON", "AMPS OFF", "VOLTS", "PF", "TEMP Live", "TEMP Neut", "CYCLE") -> (w3778:string[])
                            n2097 = Bundle By Name("Y"=w3800, "t0"=w3771) -> (w3793:waveform(dbl))  [unwired: 1 in]
                            n2098 = Bundle By Name("Y"=w3799, "t0"=w3771) -> (w3792:waveform(dbl))  [unwired: 1 in]
                            n2099 = Bundle By Name("Y"=w3798, "t0"=w3771) -> (w3791:waveform(dbl))  [unwired: 1 in]
                            n2100 = Bundle By Name("Y"=w3797, "t0"=w3771) -> (w3790:waveform(dbl))  [unwired: 1 in]
                            n2101 = Bundle By Name("Y"=w3796, "t0"=w3771) -> (w3789:waveform(dbl))  [unwired: 1 in]
                            n2102 = Bundle By Name("Y"=w3795, "t0"=w3771) -> (w3788:waveform(dbl))  [unwired: 1 in]
                            n2103 = Bundle By Name("Y"=w3794, "t0"=w3771) -> (w3787:waveform(dbl))  [unwired: 1 in]
                            n2104 = Build Array(w3793, w3792, w3791, w3790, w3789, w3788, w3787) -> (w3786:waveform(dbl)[])
                            n2105 = TDMS Write(0:w3804, 5:"TEST VALUES", 7:w3778, 9:w3786) -> (4:w3777:refnum<k34>, 6:w3776:string, 15:w3775:errorcluster)  [unwired: 2 in, 1 out]
                            n2106 = TDMS Write(0:w3777, 5:w3776, 7:"TIME", 9:w3773, 11:w3775) -> (15:w3772:errorcluster)  [unwired: 1 in, 3 out]
                            n2107 = local write "data file error"(w3772) -> ()
                          }
                        }
                      }
                    }
                  }
                }
              }
              frame #1 {
                n2108 = case shown="True" w3808 {
                  tunnel: w3812 -> [_ w3817]
                  tunnel: w3811 -> [_ w3816]
                  tunnel: w3810 -> [_ w3814]
                  tunnel: w3809 -> [_ w3813]
                  frame False {
                  }
                  frame True {
                    n2109 = local read "DISP LAB01-2"() -> (w3818:T4)
                    n2110 = local read "SIG LAB01-2"() -> (w3819:T2)
                    n2111 = local read "ON L01-2"() -> (w3815:cluster{"amps":dbl, "volts":dbl, "pf":dbl})
                    n2112 = Unbundle(w3819) -> ("AMPS"=w3825:dbl, "VOLTS"=w3823:dbl, "PF"=w3822:dbl, "Tmp Live"=w3821:dbl, "Tmp Neut"=w3824:dbl)
                    n2113 = Unbundle(w3818) -> ("CYCLE"=w3820:dbl)  [unwired: 2 out]
                    n2114 = stacked-sequence {
                      tunnel: w3825 -> [w3829 w3848]
                      tunnel: w3824 -> [_ w3847]
                      tunnel: w3823 -> [w3828 w3846]
                      tunnel: w3822 -> [w3827 w3845]
                      tunnel: w3821 -> [_ w3844]
                      tunnel: w3820 -> [_ w3843]
                      tunnel: w3817 -> [_ w3842]
                      tunnel: w3816 -> [w3830 _]
                      tunnel: w3815 -> [w3826 w3840]
                      tunnel: w3814 -> [_ w3841]
                      tunnel: w3813 -> [_ w3836]
                      frame #0 {
                        n2115 = case shown="True" w3830 {
                          tunnel: w3829 -> [_ w3835]
                          tunnel: w3828 -> [_ w3834]
                          tunnel: w3827 -> [_ w3833]
                          tunnel: w3826 -> [_ w3831]
                          frame False {
                          }
                          frame True {
                            n2116 = Bundle(cluster=w3831, "amps"=w3835, "volts"=w3834, "pf"=w3833) -> (w3832:cluster{"amps":dbl, "volts":dbl, "pf":dbl})
                            n2117 = local write "ON L01-2"(w3832) -> ()
                          }
                        }
                      }
                      frame #1 {
                        n2118 = Unbundle(w3840) -> ("amps"=w3839:dbl, "volts"=w3838:dbl, "pf"=w3837:dbl)
                        n2119 = case shown="True" w3841 {
                          tunnel: w3848 -> [_ w3880]
                          tunnel: w3847 -> [_ w3887]
                          tunnel: w3846 -> [_ _]
                          tunnel: w3845 -> [_ _]
                          tunnel: w3844 -> [_ w3886]
                          tunnel: w3843 -> [_ w3885]
                          tunnel: w3842 -> [_ w3850]
                          tunnel: w3839 -> [_ w3882]
                          tunnel: w3838 -> [_ w3881]
                          tunnel: w3837 -> [_ w3879]
                          tunnel: w3836 -> [_ w3871]
                          frame False {
                          }
                          frame True {
                            n2120 = local read "TDMS LAB01-2"() -> (w3884:refnum<k34>)
                            n2121 = Build Array(w3881) -> (w3876:dbl[])
                            n2122 = Build Array(w3879) -> (w3875:dbl[])
                            n2123 = Build Array(w3886) -> (w3874:dbl[])
                            n2124 = Build Array(w3887) -> (w3873:dbl[])
                            n2125 = Build Array(w3882) -> (w3878:dbl[])
                            n2126 = Build Array(w3880) -> (w3877:dbl[])
                            n2127 = Build Array(w3885) -> (w3872:dbl[])
                            n2128 = Build Array("AMPS ON", "AMPS OFF", "VOLTS", "PF", "TEMP Live", "TEMP Neut", "CYCLE") -> (w3855:string[])
                            n2129 = Bundle By Name("Y"=w3878, "t0"=w3871) -> (w3870:waveform(dbl))  [unwired: 1 in]
                            n2130 = Bundle By Name("Y"=w3877, "t0"=w3871) -> (w3869:waveform(dbl))  [unwired: 1 in]
                            n2131 = Bundle By Name("Y"=w3876, "t0"=w3871) -> (w3868:waveform(dbl))  [unwired: 1 in]
                            n2132 = Bundle By Name("Y"=w3875, "t0"=w3871) -> (w3867:waveform(dbl))  [unwired: 1 in]
                            n2133 = Bundle By Name("Y"=w3874, "t0"=w3871) -> (w3866:waveform(dbl))  [unwired: 1 in]
                            n2134 = Bundle By Name("Y"=w3873, "t0"=w3871) -> (w3865:waveform(dbl))  [unwired: 1 in]
                            n2135 = Bundle By Name("Y"=w3872, "t0"=w3871) -> (w3864:waveform(dbl))  [unwired: 1 in]
                            n2136 = Build Array(w3870, w3869, w3868, w3867, w3866, w3865, w3864) -> (w3863:waveform(dbl)[])
                            n2137 = TDMS Write(0:w3884, 5:"TEST VALUES", 7:w3855, 9:w3863) -> (4:w3854:refnum<k34>, 6:w3853:string, 15:w3852:errorcluster)  [unwired: 2 in, 1 out]
                            n2138 = TDMS Write(0:w3854, 5:w3853, 7:"TIME", 9:w3850, 11:w3852) -> (15:w3849:errorcluster)  [unwired: 1 in, 3 out]
                            n2139 = local write "data file error"(w3849) -> ()
                          }
                        }
                      }
                    }
                  }
                }
              }
              frame #2 {
                n2140 = case shown="True" w3888 {
                  tunnel: w3892 -> [_ w3897]
                  tunnel: w3891 -> [_ w3896]
                  tunnel: w3890 -> [_ w3894]
                  tunnel: w3889 -> [_ w3893]
                  frame False {
                  }
                  frame True {
                    n2141 = local read "DISP LAB02-1"() -> (w3898:T4)
                    n2142 = local read "SIG LAB02-1"() -> (w3899:T2)
                    n2143 = local read "ON L02-1"() -> (w3895:cluster{"amps":dbl, "volts":dbl, "pf":dbl})
                    n2144 = Unbundle(w3899) -> ("AMPS"=w3905:dbl, "VOLTS"=w3903:dbl, "PF"=w3902:dbl, "Tmp Live"=w3901:dbl, "Tmp Neut"=w3904:dbl)
                    n2145 = Unbundle(w3898) -> ("CYCLE"=w3900:dbl)  [unwired: 2 out]
                    n2146 = stacked-sequence {
                      tunnel: w3905 -> [w3909 w3928]
                      tunnel: w3904 -> [_ w3927]
                      tunnel: w3903 -> [w3908 w3926]
                      tunnel: w3902 -> [w3907 w3925]
                      tunnel: w3901 -> [_ w3924]
                      tunnel: w3900 -> [_ w3923]
                      tunnel: w3897 -> [_ w3922]
                      tunnel: w3896 -> [w3910 _]
                      tunnel: w3895 -> [w3906 w3920]
                      tunnel: w3894 -> [_ w3921]
                      tunnel: w3893 -> [_ w3916]
                      frame #0 {
                        n2147 = case shown="True" w3910 {
                          tunnel: w3909 -> [_ w3915]
                          tunnel: w3908 -> [_ w3914]
                          tunnel: w3907 -> [_ w3913]
                          tunnel: w3906 -> [_ w3911]
                          frame False {
                          }
                          frame True {
                            n2148 = Bundle(cluster=w3911, "amps"=w3915, "volts"=w3914, "pf"=w3913) -> (w3912:cluster{"amps":dbl, "volts":dbl, "pf":dbl})
                            n2149 = local write "ON L02-1"(w3912) -> ()
                          }
                        }
                      }
                      frame #1 {
                        n2150 = Unbundle(w3920) -> ("amps"=w3919:dbl, "volts"=w3918:dbl, "pf"=w3917:dbl)
                        n2151 = case shown="True" w3921 {
                          tunnel: w3928 -> [_ w3960]
                          tunnel: w3927 -> [_ w3967]
                          tunnel: w3926 -> [_ _]
                          tunnel: w3925 -> [_ _]
                          tunnel: w3924 -> [_ w3966]
                          tunnel: w3923 -> [_ w3965]
                          tunnel: w3922 -> [_ w3930]
                          tunnel: w3919 -> [_ w3962]
                          tunnel: w3918 -> [_ w3961]
                          tunnel: w3917 -> [_ w3959]
                          tunnel: w3916 -> [_ w3951]
                          frame False {
                          }
                          frame True {
                            n2152 = local read "TDMS LAB02-1"() -> (w3964:refnum<k34>)
                            n2153 = Build Array(w3961) -> (w3956:dbl[])
                            n2154 = Build Array(w3959) -> (w3955:dbl[])
                            n2155 = Build Array(w3966) -> (w3954:dbl[])
                            n2156 = Build Array(w3967) -> (w3953:dbl[])
                            n2157 = Build Array(w3962) -> (w3958:dbl[])
                            n2158 = Build Array(w3960) -> (w3957:dbl[])
                            n2159 = Build Array(w3965) -> (w3952:dbl[])
                            n2160 = Build Array("AMPS ON", "AMPS OFF", "VOLTS", "PF", "TEMP Live", "TEMP Neut", "CYCLE") -> (w3935:string[])
                            n2161 = Bundle By Name("Y"=w3958, "t0"=w3951) -> (w3950:waveform(dbl))  [unwired: 1 in]
                            n2162 = Bundle By Name("Y"=w3957, "t0"=w3951) -> (w3949:waveform(dbl))  [unwired: 1 in]
                            n2163 = Bundle By Name("Y"=w3956, "t0"=w3951) -> (w3948:waveform(dbl))  [unwired: 1 in]
                            n2164 = Bundle By Name("Y"=w3955, "t0"=w3951) -> (w3947:waveform(dbl))  [unwired: 1 in]
                            n2165 = Bundle By Name("Y"=w3954, "t0"=w3951) -> (w3946:waveform(dbl))  [unwired: 1 in]
                            n2166 = Bundle By Name("Y"=w3953, "t0"=w3951) -> (w3945:waveform(dbl))  [unwired: 1 in]
                            n2167 = Bundle By Name("Y"=w3952, "t0"=w3951) -> (w3944:waveform(dbl))  [unwired: 1 in]
                            n2168 = Build Array(w3950, w3949, w3948, w3947, w3946, w3945, w3944) -> (w3943:waveform(dbl)[])
                            n2169 = TDMS Write(0:w3964, 5:"TEST VALUES", 7:w3935, 9:w3943) -> (4:w3934:refnum<k34>, 6:w3933:string, 15:w3932:errorcluster)  [unwired: 2 in, 1 out]
                            n2170 = TDMS Write(0:w3934, 5:w3933, 7:"TIME", 9:w3930, 11:w3932) -> (15:w3929:errorcluster)  [unwired: 1 in, 3 out]
                            n2171 = local write "data file error"(w3929) -> ()
                          }
                        }
                      }
                    }
                  }
                }
              }
              frame #3 {
                n2172 = case shown="True" w3968 {
                  tunnel: w3972 -> [_ w3977]
                  tunnel: w3971 -> [_ w3976]
                  tunnel: w3970 -> [_ w3974]
                  tunnel: w3969 -> [_ w3973]
                  frame False {
                  }
                  frame True {
                    n2173 = local read "DISP LAB02-2"() -> (w3978:T4)
                    n2174 = local read "SIG LAB02-2"() -> (w3979:T2)
                    n2175 = local read "ON L02-2"() -> (w3975:cluster{"amps":dbl, "volts":dbl, "pf":dbl})
                    n2176 = Unbundle(w3979) -> ("AMPS"=w3985:dbl, "VOLTS"=w3983:dbl, "PF"=w3982:dbl, "Tmp Live"=w3981:dbl, "Tmp Neut"=w3984:dbl)
                    n2177 = Unbundle(w3978) -> ("CYCLE"=w3980:dbl)  [unwired: 2 out]
                    n2178 = stacked-sequence {
                      tunnel: w3985 -> [w3989 w4008]
                      tunnel: w3984 -> [_ w4007]
                      tunnel: w3983 -> [w3988 w4006]
                      tunnel: w3982 -> [w3987 w4005]
                      tunnel: w3981 -> [_ w4004]
                      tunnel: w3980 -> [_ w4003]
                      tunnel: w3977 -> [_ w4002]
                      tunnel: w3976 -> [w3990 _]
                      tunnel: w3975 -> [w3986 w4000]
                      tunnel: w3974 -> [_ w4001]
                      tunnel: w3973 -> [_ w3996]
                      frame #0 {
                        n2179 = case shown="True" w3990 {
                          tunnel: w3989 -> [_ w3995]
                          tunnel: w3988 -> [_ w3994]
                          tunnel: w3987 -> [_ w3993]
                          tunnel: w3986 -> [_ w3991]
                          frame False {
                          }
                          frame True {
                            n2180 = Bundle(cluster=w3991, "amps"=w3995, "volts"=w3994, "pf"=w3993) -> (w3992:cluster{"amps":dbl, "volts":dbl, "pf":dbl})
                            n2181 = local write "ON L02-2"(w3992) -> ()
                          }
                        }
                      }
                      frame #1 {
                        n2182 = Unbundle(w4000) -> ("amps"=w3999:dbl, "volts"=w3998:dbl, "pf"=w3997:dbl)
                        n2183 = case shown="True" w4001 {
                          tunnel: w4008 -> [_ w4040]
                          tunnel: w4007 -> [_ w4047]
                          tunnel: w4006 -> [_ _]
                          tunnel: w4005 -> [_ _]
                          tunnel: w4004 -> [_ w4046]
                          tunnel: w4003 -> [_ w4045]
                          tunnel: w4002 -> [_ w4010]
                          tunnel: w3999 -> [_ w4042]
                          tunnel: w3998 -> [_ w4041]
                          tunnel: w3997 -> [_ w4039]
                          tunnel: w3996 -> [_ w4031]
                          frame False {
                          }
                          frame True {
                            n2184 = local read "TDMS LAB02-2"() -> (w4044:refnum<k34>)
                            n2185 = Build Array(w4041) -> (w4036:dbl[])
                            n2186 = Build Array(w4039) -> (w4035:dbl[])
